vi "SelectionValve_go_to.vi"(8 "error in (no error)":errorcluster, 11 "VISA resource name":refnum<visa-resource-name>) -> (0 "error out":errorcluster)   [LabVIEW 2015]
uses:
  <vilib>/Instr/_visa.llb/VISA Configure Serial Port (Instr).vi
panel:
  in  "Position":string
  out "return count":u32
  # "Inject Sample"
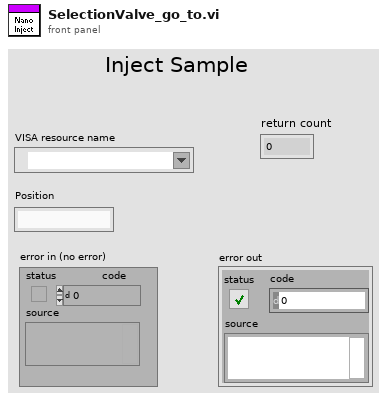
[diagram p1: front panel]
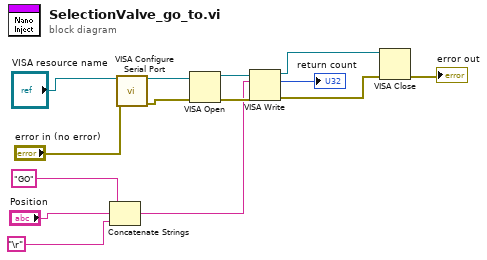
[diagram p0: block diagram]
diagram:
  n1 = Concatenate Strings("GO", "Position", "\r") -> (w1:string)
  n2 = call-poly "VISA Configure Serial Port"("VISA resource name"="VISA resource name", "error in (no error)"="error in (no error)") -> ("VISA resource name out"=w12:refnum<visa-resource-name>, "error out"=w11:errorcluster)  [unwired: 12 in]
  n3 = VISA Open(error in (no error)=w11, VISA resource name=w12) -> (VISA resource name=w14:refnum<visa-resource-name>, error out=w10:errorcluster)  [unwired: 3 in]
  n4 = VISA Write(VISA resource name=w14, write buffer=w1, error in (no error)=w10) -> (VISA resource name out=w7:refnum<visa-resource-name>, return count=→"return count":u32, error out=w8:errorcluster)
  n5 = VISA Close(VISA resource name=w7, error in (no error)=w8) -> (error out=→"error out":errorcluster)
